vi "NF WF1973_74 OUTP Scal.vi"(6 "Read(F)":bool, 7 "Select Function(Sin)":i32(ring) items=["Sinusoid", "Square", "Pulse", "Ramp", "USine", "CSine", "CFCSine", "ACSine", "SSine", "MCSine", "ONPSine", "OFPSine", "CONSine", "COFSine", "Gaussian", "Lorents", "Haversine", "HSPulse", "TPulse", "Sinc", "ERise", "Efall", "Solstep", "Doscillation", "OSurge", "PSurge", "TOffset", "HSEPulse", "BRRamp", "USER"], 8 "error in (no error)":errorcluster caption="Error IN", 9 "Scale(FS)":u16(ring)=1 items=["PFS", "FS", "MFS"], 10 "Ch(Ch1)":bool, 11 "VISAsession":refnum<visa-resource-name>) -> (0 "error out":errorcluster caption="Error OUT", 2 "Query Scale":string, 3 "CopyVISAsession":refnum<visa-resource-name>)   [LabVIEW 2010]
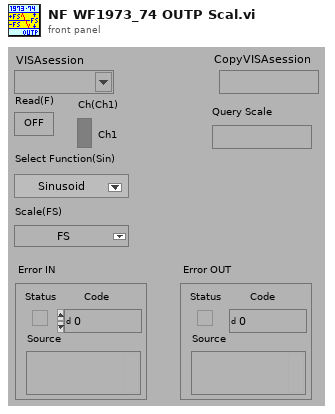
[diagram p1: front panel]
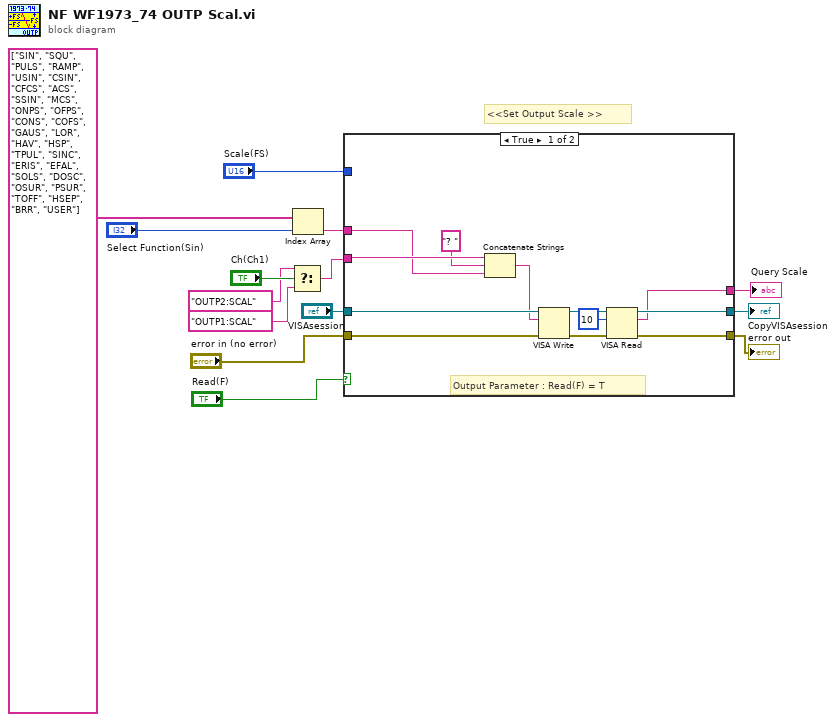
[diagram p0: block diagram]
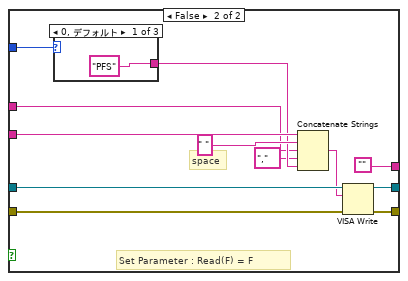
[diagram p2: hidden frame]
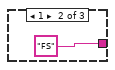
[diagram p3: hidden frame]
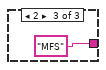
[diagram p4: hidden frame]
diagram:
  # "<<Set Output Scale >>"
  n1 = Select(t="OUTP2:SCAL" ("文字列"), s="Ch(Ch1)", f="OUTP1:SCAL" ("文字列")) -> (s? t:f=w7:string)
  n2 = Index Array(array=string[] ["SIN", "SQU", "PULS", "RAMP", "USIN", "CSIN", "CFCS", "ACS", "SSIN", "MCS", "ONPS", "OFPS", "CONS", "COFS", "GAUS", "LOR", "HAV", "HSP", "TPUL", "SINC", "ERIS", "EFAL", "SOLS", "DOSC", "OSUR", "PSUR", "TOFF", "HSEP", "BRR", "USER"] ("配列"), index="Select Function(Sin)") -> (element=w1:string)
  n3 = case shown="TRUE" "Read(F)" {
    tunnel: "VISAsession" -> [w26 w38]
    tunnel: [w23 w36] -> w13
    tunnel: [w22 w37] -> w12
    tunnel: "error in (no error)" -> [w21 w32]
    tunnel: w7 -> [w17 w33]
    tunnel: [w18 ""] -> w9
    tunnel: "Scale(FS)" -> [_ w31]
    tunnel: w1 -> [w15 w28]
    frame True {
      # "Output Parameter : Read(F) = T"
      n4 = Concatenate Strings(w17, "? " ("形式文字列"), w15) -> (w19:string)
      n5 = VISA Write(VISA resource name=w26, write buffer=w19, error in (no error)=w21) -> (VISA resource name out=w24:refnum<visa-resource-name>, error out=w25:errorcluster)  [unwired: 1 out]
      n6 = VISA Read(VISA resource name=w24, byte count=u32 10 ("バイトカウント（0）"), error in (no error)=w25) -> (VISA resource name out=w23:refnum<visa-resource-name>, read buffer=w18:string, error out=w22:errorcluster)  [unwired: 1 out]
    }
    frame False {
      # "space"
      # "Set Parameter : Read(F) = F"
      n7 = case shown="0, デフォルト" w31 {
        tunnel: ["PFS" ("文字列") "FS" ("文字列") "MFS" ("文字列")] -> w29
        frame 0, Default {
        }
        frame 1 {
        }
        frame 2 {
        }
      }
      n8 = Concatenate Strings(w33, " ", w28, "," ("文字列"), w29) -> (w35:string)
      n9 = VISA Write(VISA resource name=w38, write buffer=w35, error in (no error)=w32) -> (VISA resource name out=w36:refnum<visa-resource-name>, error out=w37:errorcluster)  [unwired: 1 out]
    }
  }
  "error out" <- w12
  "CopyVISAsession" <- w13
  "Query Scale" <- w9
